vi "update.properties.vi"(8 "error in":errorcluster, 10 "Properties":map{string, string}(c390), 11 "asset in":refnum<class "asset.lvclass">) -> (0 "error out":errorcluster, 3 "asset out":refnum<class "asset.lvclass">)   [LabVIEW 2020, in "asset.lvclass"]
uses:
  asset.lvclass
  Nominal Client/Nominal Client.lvclass
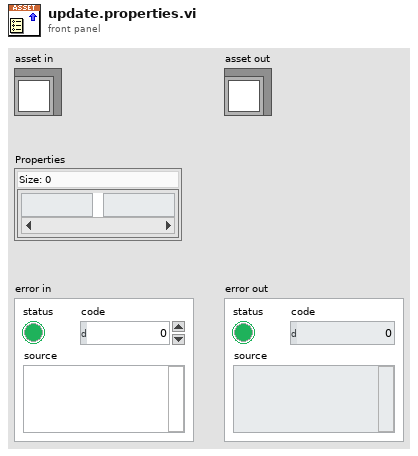
[diagram p1: front panel]
types:
  T1 = typedef "dataScopes.lvlib/links.ctl" = cluster{"URL":string, "Title":string}[]
  T2 = typedef "dataScopes.lvlib/data_scopes.ctl" = T3[]
  T3 = typedef "dataScopes.lvlib/data_scope.ctl" = cluster{"dataScopeName":string, "dataSource":T4, "seriesTags":map{string, string}, "offset":T6}
  T4 = typedef "dataScopes.lvlib/data_source.ctl" = cluster{"type":T5, "rid":string}
  T5 = typedef "dataScopes.lvlib/type.ctl" = enum16{"dataset", "connection", "logSet", "video"}
  T6 = typedef "dataScopes.lvlib/offset.ctl" = cluster{"seconds":i32, "nanos":i32, "picos":i32}
  T7 = cluster{"rid":string, "title":string, "properties":refnum<class "properties.lvclass">, "labels":refnum<class "labels.lvclass">, "Links":T1, "datascopes":T2, "createdAt":timestamp, "updatedAt":timestamp, "attachments":refnum<class "labels.lvclass">, "isStaged":bool, "isArchived":bool, "description":string, "createdBy":string, "type":string}
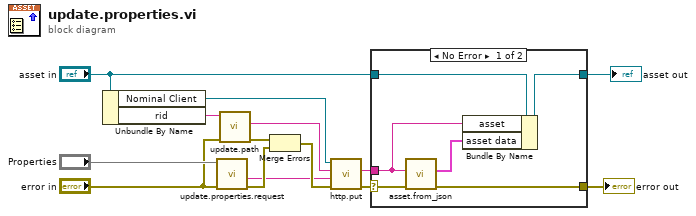
[diagram p0: block diagram]
diagram:
  n1 = Unbundle By Name("asset in") -> ("Nominal Client"=w14:refnum<class "Nominal Client.lvclass">, "rid"=w11:string)
  n2 = call "update.properties.request.vi"("error in"="error in", "properties"="Properties") -> ("error out"=w2:errorcluster, "Request"=w1:string)  [unwired: 8 in]
  n3 = call "update.path.vi"("error in"="error in", "Asset RID"=w11) -> ("error out"=w9:errorcluster, "Path"=w10:string)  [unwired: 8 in]
  n4 = Merge Errors(w9, w2) -> (w8:errorcluster)
  n5 = call "http.put.vi"("error in"=w8, "Body"=w1, "Path"=w10, "Nominal Client in"=w14) -> ("error out"=w13:errorcluster, "Response"=w12:string)  [unwired: 5 in, 1 out]
  n6 = case shown="No Error" w13 {
    selector: w13 -> [w20 w22]
    tunnel: [w19 w22] -> w6
    tunnel: "asset in" -> [w18 w21]
    tunnel: w12 -> [w16 _]
    tunnel: [w15 w21] -> w7
    frame No Error {
      n7 = call "asset.from_json.vi"("error in"=w20, "asset"=w16) -> ("error out"=w19:errorcluster, "Asset Data"=w17:T7)  [unwired: 8 in]
      n8 = Bundle By Name(cluster=w18, "asset"=w16, "asset data"=w17) -> (w15:refnum<class "asset.lvclass">)
    }
    frame Error {
    }
  }
  "asset out" <- w7
  "error out" <- w6
